vi "Update State.vi"(8 "error in (no error)":errorcluster, 11 "LFCSimShutt in":refnum<class "LFCSimShutt.lvclass">) -> (0 "error out":errorcluster, 3 "LFCSimShutt out":refnum<class "LFCSimShutt.lvclass">)   [LabVIEW 2016]
uses:
  LFCSimShutt.lvclass
  Controls/Shutter States.ctl
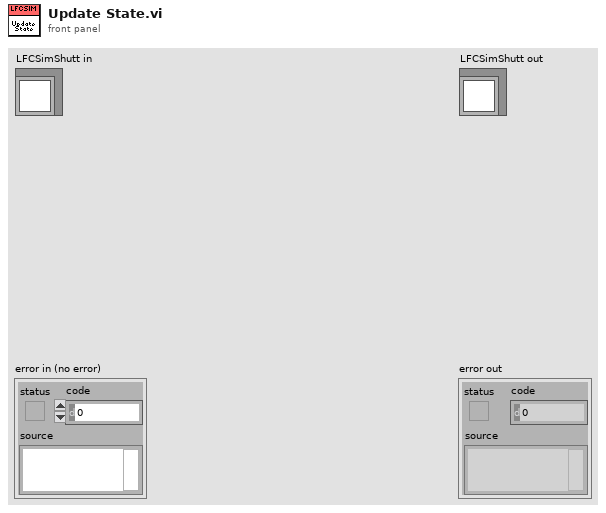
[diagram p1: front panel]
types:
  T1 = typedef "Shutter States.ctl" = enum16{"Open", "Close", "Wait", "Off", "Arm", "Idle"}
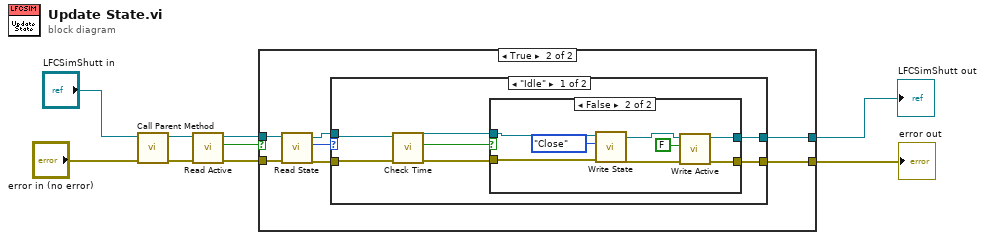
[diagram p0: block diagram]
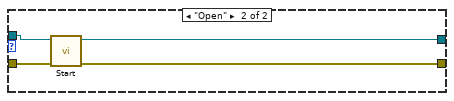
[diagram p4: hidden frame]
diagram:
  n1 = call-parent "Call Parent Method"("error in (no error)"="error in (no error)", "UniStableShutter in"="LFCSimShutt in") -> ("error out"=w6:errorcluster, "UniStableShutter out"=w7:refnum<class "LFCSimShutt.lvclass">)  [unwired: 8 in]
  n2 = call-dynamic "Read Active.vi"("error in (no error)"=w6, "Integrator in"=w7) -> ("error out"=w3:errorcluster, "Active"=w5:bool, "Integrator out"=w4:refnum<class "LFCSimShutt.lvclass">)  [unwired: 7 in]
  n3 = case shown="True" w5 {
    tunnel: w4 -> [w11 w18]
    tunnel: w3 -> [w10 w17]
    tunnel: [w11 w13] -> w2
    tunnel: [w10 w12] -> w1
    frame False {
    }
    frame True {
      n4 = call-dynamic "Read State.vi"("error in (no error)"=w17, "Shutter in"=w18) -> ("error out"=w14:errorcluster, "State"=w16:T1, "Shutter out"=w15:refnum<class "LFCSimShutt.lvclass">)  [unwired: 7 in]
      n5 = case shown="\"Idle\"" w16 {
        tunnel: w15 -> [w25 w39]
        tunnel: w14 -> [w24 w38]
        tunnel: [w23 w37] -> w13
        tunnel: [w22 w36] -> w12
        frame "Idle" {
          n6 = call-dynamic "Check Time.vi"("error in (no error)"=w24, "Integrator in"=w25) -> ("error out"=w19:errorcluster, "On"=w21:bool, "Integrator out"=w20:refnum<class "LFCSimShutt.lvclass">)  [unwired: 7 in]
          n7 = case shown="False" w21 {
            tunnel: w20 -> [w26 w35]
            tunnel: w19 -> [w27 w34]
            tunnel: [w26 w31] -> w23
            tunnel: [w27 w30] -> w22
            frame True {
            }
            frame False {
              n8 = call-dynamic "Write State.vi"("error in (no error)"=w34, "State"=Shutter_States."Close", "UniStableShutter in"=w35) -> ("error out"=w29:errorcluster, "UniStableShutter out"=w32:refnum<class "LFCSimShutt.lvclass">)  [unwired: 7 in]
              n9 = call-dynamic "Write Active.vi"("error in (no error)"=w29, "Active"=FALSE, "Integrator in"=w32) -> ("error out"=w30:errorcluster, "Integrator out"=w31:refnum<class "LFCSimShutt.lvclass">)  [unwired: 7 in]
            }
          }
        }
        frame "Open" {
          n10 = call-dynamic "Start.vi"("error in (no error)"=w38, "Integrator in"=w39) -> ("error out"=w36:errorcluster, "Integrator out"=w37:refnum<class "LFCSimShutt.lvclass">)  [unwired: 8 in]
        }
      }
    }
  }
  "error out" <- w1
  "LFCSimShutt out" <- w2
